vi "API_Unblock.vi"(1 "Argument List In":string[](array[string])) -> (0 "Argument List Out":string[](array[string]))   [LabVIEW 2011]
doc: "This VI, when called inside a currently running API function, will unblock execution. For example, if used within an API function to set a temperature, the user would continuously check the current temperature, and when a stable temperature is been reached, call this VI to halt execution of the temperature API function and continue execution of the growth sequence."
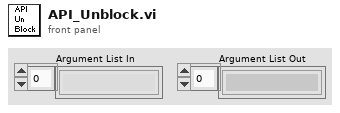
[diagram p1: front panel]
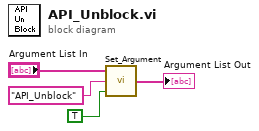
[diagram p0: block diagram]
diagram:
  n1 = call "Set_Argument.vi"("Enable"=TRUE, "Argument"="API_Unblock", "Argument List In"="Argument List In") -> ("Argument List Out"=→"Argument List Out":string[])
